vi "Recipe_Type.vi"() -> ()   [LabVIEW 2017]
panel:
  out "Recipe_name":string
  out "ST_1_ROLLER":bool
  out "ST_1_SCREW":bool
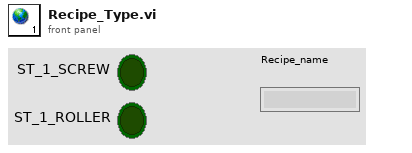
[diagram p1: front panel]
diagram:
